vi "TcpIPTest.vi"() -> ()   [LabVIEW 2011]
panel:
  out "整理后的数据":string[](array[string])
  in  "停止":bool
  out "数据输出":string
  in  "远程端口或服务名称":u16=2000
  in  "地址":string="192.168.0.4"
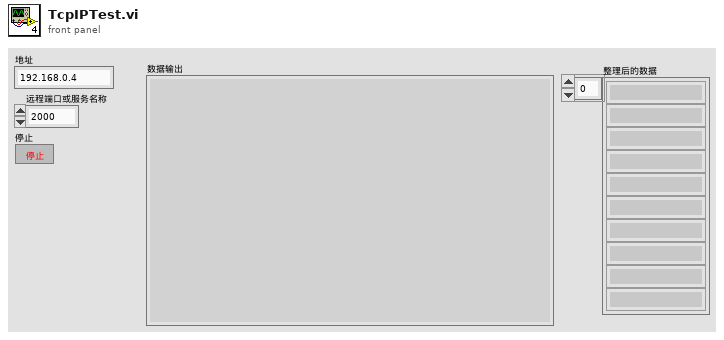
[diagram p1: front panel]
types:
  T1 = enum16{"Standard", "Buffered", "CRLF", "Immediate"}
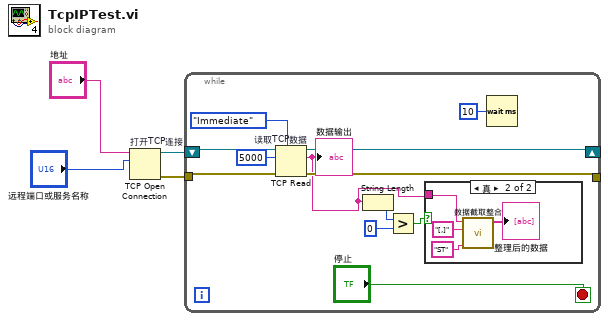
[diagram p0: block diagram]
diagram:
  n1 = TCP Open Connection "打开TCP连接"(address="地址", remote port or service name="远程端口或服务名称") -> (connection ID=w2:refnum<k5>, error out=w1:errorcluster)  [unwired: 3 in]
  n2 = while {
    shift-right: [w13] -> _
    shift-left: w2 -> [w16]
    tunnel: w1 -> [w15]
    tunnel: [w12] -> _
    stop <- "停止" stop-if-true
    n3 = TCP Read "读取TCP数据"(connection ID=w16, bytes to read=5000 ("读取的字节"), error in (no error)=w15, 7:T1."Immediate" ("模式（标准）")) -> (connection ID out=w13:refnum<k5>, data out=w6:string, error out=w12:errorcluster)  [unwired: 1 in]
    "数据输出" <- w6
    n4 = String Length(string=w6) -> (length=w9:i32)
    n5 = Greater?(x=w9, y=0) -> (0:w7:bool)
    n6 = case shown="真" w7 {
      tunnel: w6 -> [_ w20]
      frame False {
      }
      frame True {
        n7 = call "数据截取整合.vi"("Input Data"=w20, "正则表达式"="[,]", "起始元素"="ST") -> ("整理后的数据"=→"整理后的数据":string[])  [unwired: 6 in]
      }
    }
    n8 = Wait (ms)(milliseconds to wait=u32 10 ("等待时间（毫秒）")) -> ()  [unwired: 1 out]
  }
